vi "create folder if not exists.vi"(8 "error in":errorcluster, 11 "Directory Path":path) -> (0 "error out":errorcluster, 3 "Directory Path":path)   [LabVIEW 2020, in "Reusable Library.lvlib"]
uses:
  Reusable Library.lvlib
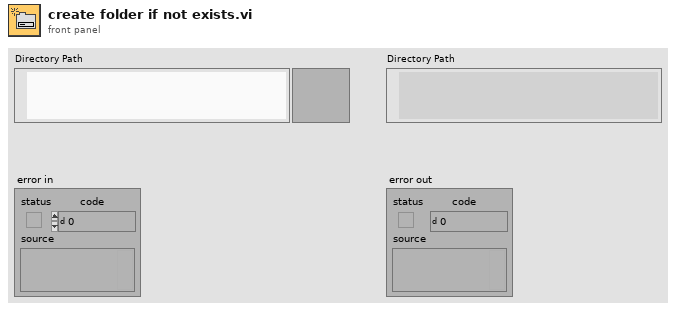
[diagram p1: front panel]
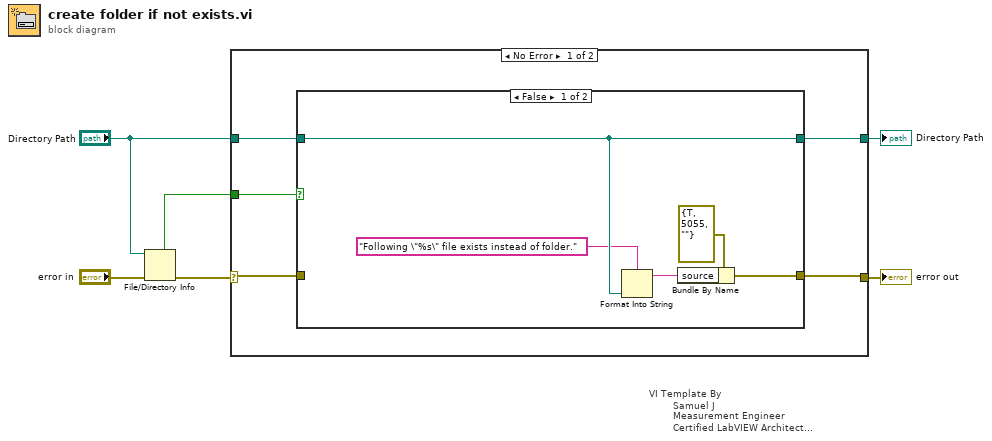
[diagram p0: block diagram]
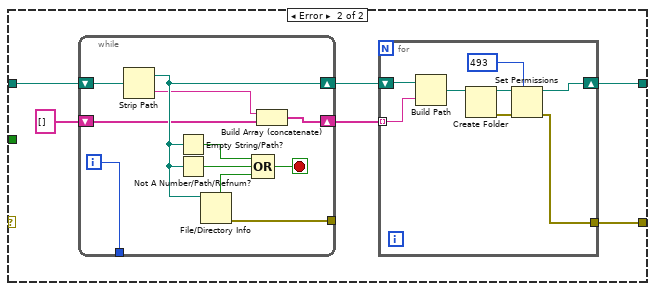
[diagram p3: hidden frame]
diagram:
  n1 = File/Directory Info(path="Directory Path", error in="error in") -> (directory=w1:bool, error out=w2:errorcluster)  [unwired: 5 out]
  n2 = case "VI Template By\n        Samuel J\n        Measurement Engineer\n        Certified LabVIEW Architect\n        Vestas Technology R&D, Chennai" shown="No Error" w2 {
    selector: w2 -> [w9 _]
    tunnel: [w10 w20] -> w6
    tunnel: "Directory Path" -> [w7 w24]
    tunnel: [w8 w23] -> w5
    tunnel: w1 -> [w11 _]
    frame No Error {
      n3 = case shown="False" w11 {
        tunnel: [w12 w18] -> w10
        tunnel: w9 -> [_ w18]
        tunnel: [w16 w17] -> w8
        tunnel: w7 -> [w16 w17]
        frame False {
          n4 = Format Into String(format string="Following \"%s\" file exists instead of folder.", w16) -> (resulting string=w14:string)  [unwired: 2 in, 1 out]
          n5 = Bundle By Name(cluster=errorcluster {"status"=TRUE, "code"=5055, "source"=""} ("error IO"), "source"=w14) -> (w12:errorcluster)
        }
        frame True {
        }
      }
    }
    frame Error {
      n6 = while {
        shift-right: [w32] -> w21
        shift-left: w24 -> [w35]
        tunnel: [w29] -> _
        tunnel: [w28] -> _
        shift-right: [w25] -> w22
        shift-left: string[] [] -> [w26]
        i -> [w28]
        stop <- w30 stop-if-true
        n7 = Strip Path(path=w35) -> (stripped path=w32:path, name=w27:string)
        n8 = Empty String/Path?(string/path=w32) -> (empty?=w34:bool)
        n9 = Not A Number/Path/Refnum?(number/path/refnum=w32) -> (NaN/Path/Refnum?=w33:bool)
        n10 = File/Directory Info(path=w32) -> (directory=w31:bool, error out=w29:errorcluster)  [unwired: 1 in, 5 out]
        n11 = Compound Arithmetic op=OR(w34, w33, w31) -> (w30:bool)
        n12 = Build Array (concatenate)(w27, w26) -> (w25:string[])
      }
      n13 = for {
        tunnel: w22 -> [w43] mode=indexing
        shift-right: [w40] -> w23
        shift-left: w21 -> [w42]
        tunnel: [w36] -> w20
        n14 = Build Path(base path=w42, name or relative path=w43) -> (appended path=w41:path)
        n15 = Create Folder(path (use dialog)=w41) -> (created path=w39:path, error out=w38:errorcluster)  [unwired: 1 in, 2 out]
        n16 = Set Permissions(7:i16 493 ("permissions (0755)"), 8:w38, 11:w39) -> (0:w36:errorcluster, 3:w40:path)  [unwired: 2 out]
      }
    }
  }
  "Directory Path" <- w5
  "error out" <- w6
